vi "New Standard Command.vi"(0 "RFFE Standard Command in":refnum<class "RFFE Standard Command.lvclass">, 1 "Alias":string, 5 "Slave Address":T2=12 format="%02x", 7 "Register Address":T3 format="%02x", 9 "Register Data":T1 format="%02x", 11 "error in (no error)":errorcluster) -> (4 "RFFE Standard Command out":refnum<class "RFFE Standard Command.lvclass">, 15 "error out":errorcluster)   [LabVIEW 2018, in "MIPI RFFE API.lvlib" / "RFFE Standard Command.lvclass"]
uses:
  RFFE Standard Command.lvclass
  C:/Users/semoore/Projects/mipi-rffe-labview-oop/Command/RFFE Command.lvclass
  Register Address.ctl
  Slave Address.ctl
  Register Data.ctl
  RFFE Standard Command.lvclass/RFFE Standard Command.ctl
  Command/RFFE Command.lvclass
  MIPI RFFE API.lvlib
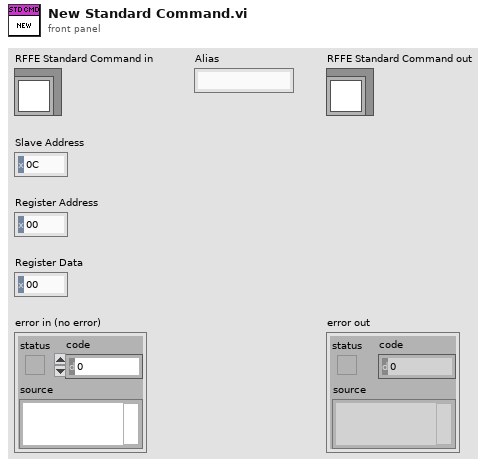
[diagram p1: front panel]
types:
  T1 = typedef "MIPI RFFE API.lvlib/Register Data.ctl" = u8
  T2 = typedef "MIPI RFFE API.lvlib/Slave Address.ctl" = u8
  T3 = typedef "MIPI RFFE API.lvlib/Register Address.ctl" = u16
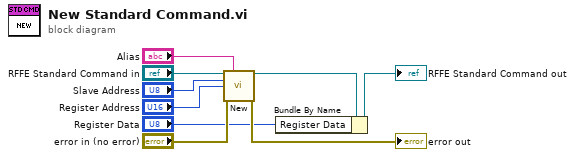
[diagram p0: block diagram]
diagram:
  n1 = call "New.vi"("RFFE Command in"="RFFE Standard Command in", "Alias"="Alias", "Slave Address"="Slave Address", "Register Address"="Register Address", "error in (no error)"="error in (no error)") -> ("RFFE Command out"=w1:refnum<class "RFFE Standard Command.lvclass">, "error out"=→"error out":errorcluster)  [unwired: 9 in]
  n2 = Bundle By Name(cluster=w1, "Register Data"="Register Data") -> (→"RFFE Standard Command out":refnum<class "RFFE Standard Command.lvclass">)
